vi "Insert Multiple into Object.vi"(5 "Item Names":string[](array[string]), 6 "Object Path":string, 7 "error in (no error)":errorcluster, 8 "JSON to Insert":string[](array[string]), 9 "Object Offset":i32, 10 "JSON in":string="{}") -> (0 "error out":errorcluster, 1 "Replaced":bool, 3 "<JSON>":string)   [LabVIEW 2013, in "JSONtext.lvlib"]
doc: "Insert multiple items into a JSON Object specified by the Object Path"
uses:
  JSONtext.lvlib
  String Subset.vi
  <userlib>/_OpenG.lib/string/string.llb/Trim Whitespace (String)__ogtk.vi
  Find Item Locations by Path.vi
  support/JSONtext support.lvlib
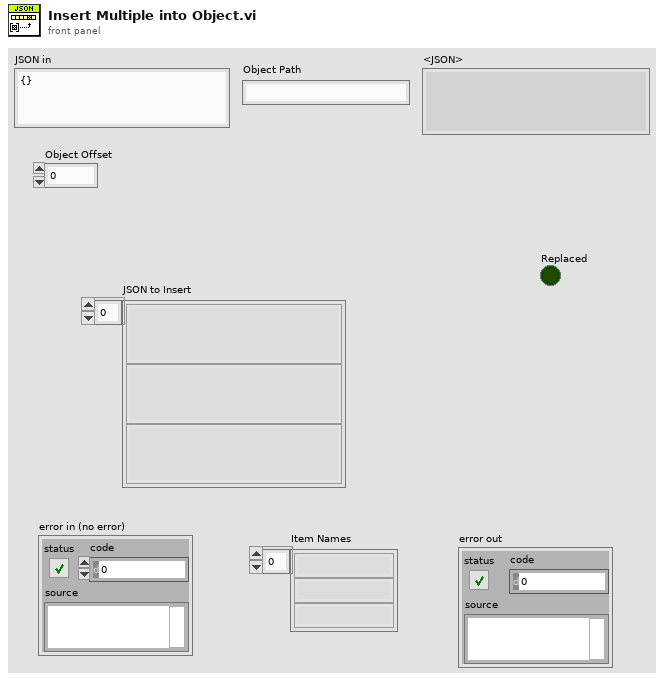
[diagram p1: front panel]
types:
  T1 = typedef "JSONtext.lvlib/Found Items.ctl" = cluster{"Item offset":i32, "Offset past Item":i32, "Name offset":i32, "Offset past Name":i32, "Found":bool, "Empty Object":bool}
  T2 = cluster{"Item":T1, "<JSON>":string, "JSON to Insert":string}
  T3 = cluster{"Item":T1, "<JSON>":string, "JSON to Insert":string}[]
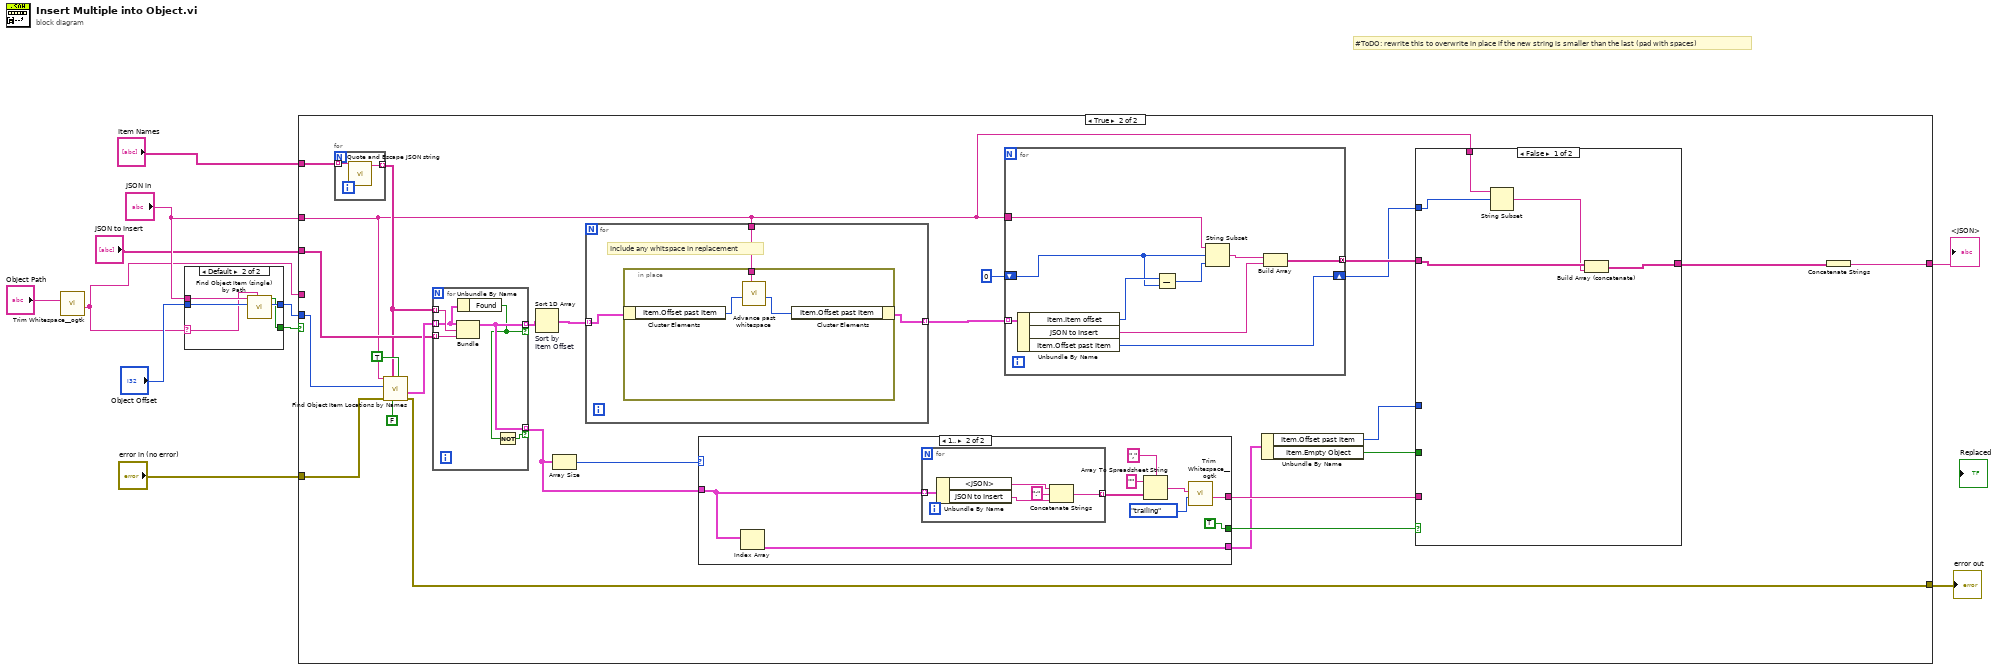
[diagram p0: block diagram]
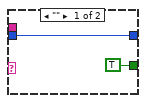
[diagram p2: hidden frame]
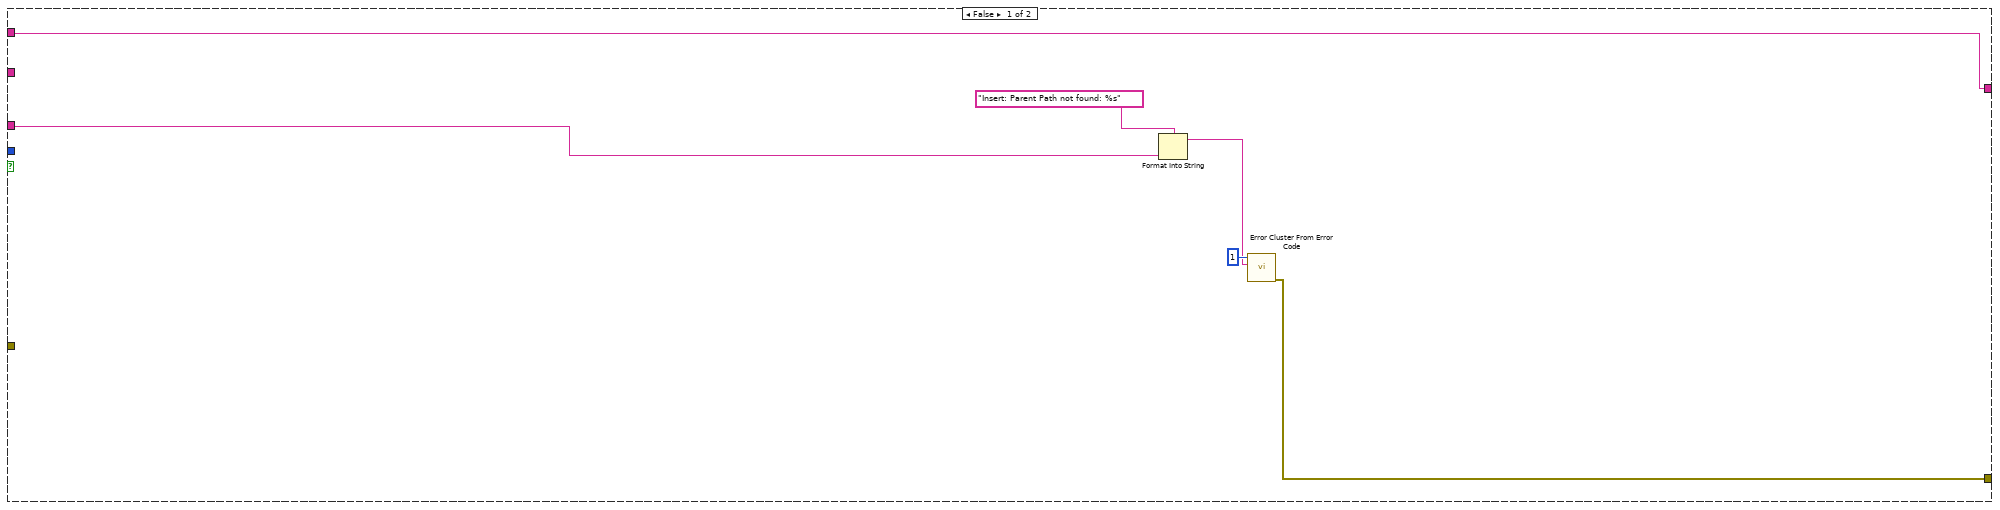
[diagram p3: hidden frame]
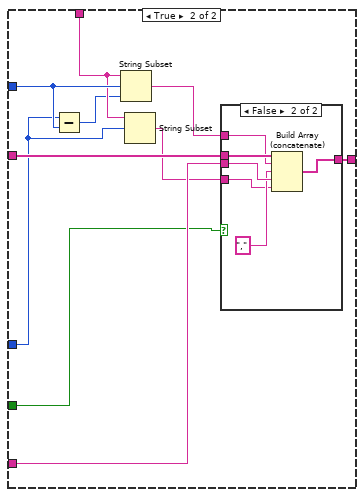
[diagram p4: hidden frame]
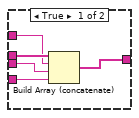
[diagram p5: hidden frame]
diagram:
  # "#ToDO: rewrite this to overwrite in place if the new string is smaller than the last (pad with spaces)"
  n1 = call-poly <userlib>:"Trim Whitespace__ogtk.vi"("String in"="Object Path") -> ("String out"=w1:string)  [unwired: 6 in]
  n2 = case shown="Default" w1 {
    selector: w1 -> [_ w14]
    tunnel: "JSON in" -> [_ w18]
    tunnel: "Object Offset" -> [w13 w17]
    tunnel: [w13 w16] -> w7
    tunnel: [TRUE ("Found") w15] -> w6
    frame "" {
    }
    frame Default {
      n3 = call "Find Object Item (single) by Path.vi"("Item Path"=w14, "Starting Offset"=w17, "JSON"=w18) -> ("Item offset"=w16:i32, "Found"=w15:bool)  [unwired: 5 in, 2 out]
    }
  }
  n4 = case shown="True" w6 {
    tunnel: "JSON to Insert" -> [_ w40]
    tunnel: "error in (no error)" -> [_ w49]
    tunnel: [w23 w48] -> w10
    tunnel: "JSON in" -> [w24 w25]
    tunnel: w7 -> [_ w47]
    tunnel: "Item Names" -> [_ w46]
    tunnel: [w24 w32] -> w3
    tunnel: w1 -> [w19 _]
    frame False {
      n5 = Format Into String(format string="Insert: Parent Path not found: %s" ("error message (\"\")"), w19) -> (resulting string=w21:string)  [unwired: 2 in, 1 out]
      n6 = call <vilib>:"Error Cluster From Error Code.vi"("error message (\"\")"=w21, "error code (0)"=1) -> ("error out"=w23:errorcluster)  [unwired: 7 in]
    }
    frame True {
      n7 = for {
        tunnel: w46 -> [w112] mode=indexing
        tunnel: [w111] -> w38 mode=indexing
        n8 = call "Quote and Escape JSON string.vi"("Plain Text"=w112) -> ("<JSON>"=w111:string)  [unwired: 10 in]
      }
      n9 = call "Find Object Item Locations by Names.vi"("Insertion point if not found"=TRUE, "Only return first found"=FALSE, "Item Names <JSON>"=w38, "error in (no error)"=w49, "Object Offset"=w47, "JSON"=w25) -> ("error out"=w48:errorcluster, "Items"=w42:T1[])  [unwired: 4 in]
      n10 = for {
        tunnel: [w98] -> w43 mode=indexing if=w96
        tunnel: w42 -> [w99] mode=indexing
        tunnel: w38 -> [w101] mode=indexing
        tunnel: w40 -> [w100] mode=indexing
        tunnel: [w98] -> w37 mode=indexing if=w97
        n11 = Bundle("Item"=w99, "<JSON>"=w101, "JSON to Insert"=w100) -> (w98:T2)  [unwired: 1 in]
        n12 = Unbundle By Name(w99) -> ("Found"=w96:bool)
        n13 = Not(x=w96) -> (.not. x?=w97:bool)
      }
      n14 = Sort 1D Array "Sort by \nItem Offset"(array=w43) -> (sorted array=w41:T3)
      n15 = Array Size(array=w37) -> (size(s)=w36:i32)
      n16 = for {
        tunnel: w41 -> [w92] mode=indexing
        tunnel: [w91] -> w39 mode=indexing
        tunnel: w25 -> [w90]
        # "Include any whitspace in replacement"
        n17 = in-place {
          in-place-border: w90 -> [w94]
          n18 = in-place-cluster #1(w92) -> ("Item.Offset past Item"=w95:i32)
          n19 = call "Advance past whitespace.vi"("JSON"=w94, "Offset"=w95) -> ("Offset of first non-whitespace"=w93:i32)  [unwired: 8 in, 1 out]
          n20 = in-place-cluster #1("Item.Offset past Item"=w93) -> (w91:T2)
        }
      }
      n21 = case shown="1.." w36 {
        tunnel: w37 -> [_ w79]
        tunnel: [_ w78] -> w29
        tunnel: [_ w77] -> w33
        tunnel: [_ TRUE] -> w35
        frame 0, Default {
        }
        frame 1.. {
          n22 = Index Array(array=w79) -> (element=w78:T2)  [unwired: 1 in]
          n23 = for {
            tunnel: w79 -> [w89] mode=indexing
            tunnel: [w85] -> w84 mode=indexing
            n24 = Unbundle By Name(w89) -> ("<JSON>"=w88:string, "JSON to Insert"=w87:string)
            n25 = Concatenate Strings(w88, ":" ("string"), w87) -> (w85:string)
          }
          n26 = Array To Spreadsheet String(delimiter (Tab)=",", array=w84, 3:"" ("format string")) -> (spreadsheet string=w81:string)
          n27 = call-poly <userlib>:"Trim Whitespace__ogtk.vi"("Remove (leading and trailing)"=enum16{"leading", "trailing", "both"}."trailing", "String in"=w81) -> ("String out"=w77:string)  [unwired: 5 in]
        }
      }
      n28 = for {
        tunnel: w25 -> [w108]
        tunnel: w39 -> [w110] mode=indexing
        tunnel: [w106] -> w34 mode=concatenating
        shift-right: [w105] -> w30
        shift-left: 0 ("Offset\nAdjustment") -> [w103]
        n29 = Unbundle By Name(w110) -> ("Item.Item offset"=w104:i32, "JSON to Insert"=w107:string, "Item.Offset past Item"=w105:i32)
        n30 = Subtract(x=w104, y=w103) -> (x-y=w102:i32)
        n31 = String Subset(string=w108, offset (0)=w103, length (rest)=w102) -> (substring=w109:string)
        n32 = Build Array(w109, w107) -> (w106:string[])
      }
      n33 = Unbundle By Name(w29) -> ("Item.Offset past Item"=w27:i32, "Item.Empty Object"=w28:bool)
      n34 = case shown="False" w35 {
        tunnel: w34 -> [w54 w64]
        tunnel: w33 -> [_ w62]
        tunnel: [w51 w63] -> w26
        tunnel: w25 -> [w53 w59]
        tunnel: w30 -> [w52 w60]
        tunnel: w28 -> [_ w61]
        tunnel: w27 -> [_ w55]
        frame False {
          n35 = String Subset(string=w53, offset (0)=w52) -> (substring=w50:string)  [unwired: 1 in]
          n36 = Build Array (concatenate)(w54, w50) -> (w51:string[])
        }
        frame True {
          n37 = Subtract(x=w55, y=w60) -> (x-y=w58:i32)
          n38 = String Subset(string=w59, offset (0)=w60, length (rest)=w58) -> (substring=w57:string)
          n39 = String Subset(string=w59, offset (0)=w55) -> (substring=w56:string)  [unwired: 1 in]
          n40 = case shown="False" w61 {
            tunnel: w64 -> [w69 w75]
            tunnel: w62 -> [w68 w74]
            tunnel: [w67 w73] -> w63
            tunnel: w57 -> [w65 w70]
            tunnel: w56 -> [w66 w71]
            frame True {
              n41 = Build Array (concatenate)(w69, w65, w68, w66) -> (w67:string[])
            }
            frame False {
              n42 = Build Array (concatenate)(w75, w70, "," ("element"), w74, w71) -> (w73:string[])
            }
          }
        }
      }
      n43 = Concatenate Strings(w26) -> (w32:string)
    }
  }
  "<JSON>" <- w3
  "error out" <- w10
